vi "Tegam4040_Multi_Driver.vi"(9 "Input":dbl, 10 "Function":T1(ring), 11 "VISA Tegam4040":refnum<visa-resource-name>="PXI4::12::INSTR") -> (0 "error out":errorcluster)   [LabVIEW 2010]
uses:
  <instrlib>/Tegam4040/Tegam4040.lvlib
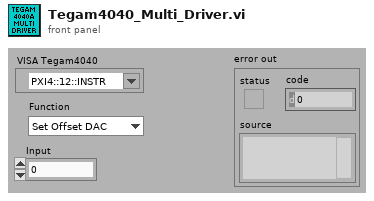
[diagram p1: front panel]
types:
  T1 = enum16{"Set Offset DAC", "Set Coupling (0=DC, 1=AC)", "Set Input (0=1M,1=50ohms)", "Set Atten (0-3=Open,1,10,100)", "Set Gain (0-2=1,10,100)"}
  T2 = enum16{"Attenuator Stage open", "Attenuation of 1", "Attenuation of 10", "Attenuation of 100"}
  T3 = enum16{"Disable Calibration", "Enable Calibration"}
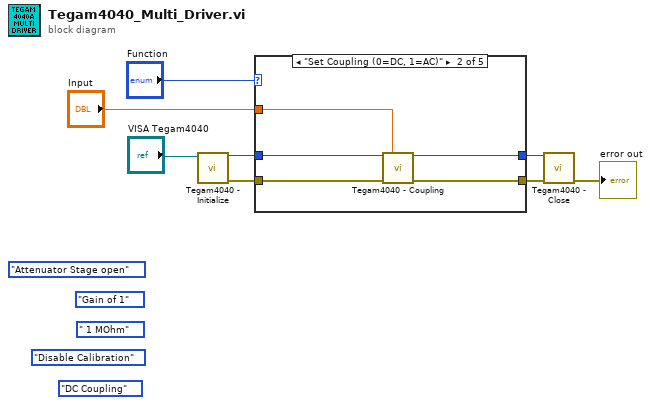
[diagram p0: block diagram]
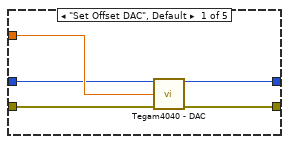
[diagram p2: hidden frame]
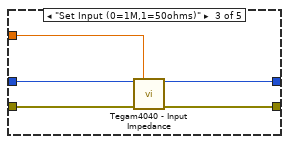
[diagram p3: hidden frame]
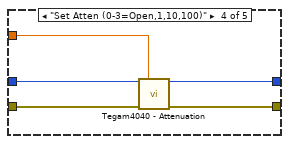
[diagram p4: hidden frame]
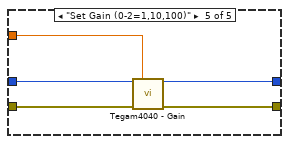
[diagram p5: hidden frame]
diagram:
  (unwired) T2."Attenuator Stage open" ("Attenuation")
  (unwired) enum16{"Gain of 1", "Gain of 10", "Gain of 100"}."Gain of 1" ("Gain")
  (unwired) enum16{" 1 MOhm", "50 Ohm"}." 1 MOhm" ("Input Impedance")
  (unwired) T3."Disable Calibration" ("Calibration")
  (unwired) enum16{"DC Coupling", "AC Coupling"}."DC Coupling" ("Coupling")
  n1 = call <instrlib>:"Tegam4040 - Initialize.vi"("VISA Tegam4040"="VISA Tegam4040") -> ("error out"=w7:errorcluster, "Instrument Session Handle"=w2:u32)  [unwired: 9 in]
  n2 = case shown="\"Set Coupling (0=DC, 1=AC)\"" "Function" {
    tunnel: w7 -> [w13 w17 w22 w28 w32]
    tunnel: [w12 w18 w23 w27 w33] -> w6
    tunnel: "Input" -> [w11 w14 w19 w24 w29]
    tunnel: w2 -> [w10 w16 w20 w26 w31]
    tunnel: [w9 w15 w21 w25 w30] -> w1
    frame "Set Offset DAC", Default {
      n3 = call <instrlib>:"Tegam4040 - DAC.vi"("Instrument Session Handle In"=w10, "DAC"=w11, "error in (no error)"=w13) -> ("Instrument Session Handle Out (dupl)"=w9:u32, "error out"=w12:errorcluster)  [unwired: 11 in]
    }
    frame "Set Coupling (0=DC, 1=AC)" {
      n4 = call <instrlib>:"Tegam4040 - Coupling.vi"("Instrument Session Handle In"=w16, "Coupling"=w14, "error in (no error)"=w17) -> ("Instrument Session Handle Out (dupl)"=w15:u32, "error out"=w18:errorcluster)  [unwired: 11 in]
    }
    frame "Set Input (0=1M,1=50ohms)" {
      n5 = call <instrlib>:"Tegam4040 - Input Impedance.vi"("Instrument Session Handle In"=w20, "Input Impedance"=w19, "error in (no error)"=w22) -> ("Instrument Session Handle Out (dupl)"=w21:u32, "error out"=w23:errorcluster)  [unwired: 11 in]
    }
    frame "Set Atten (0-3=Open,1,10,100)" {
      n6 = call <instrlib>:"Tegam4040 - Attenuation.vi"("Instrument Session Handle In"=w26, "Attenuation"=w24, "error in (no error)"=w28) -> ("Instrument Session Handle Out (dupl)"=w25:u32, "error out"=w27:errorcluster)  [unwired: 11 in]
    }
    frame "Set Gain (0-2=1,10,100)" {
      n7 = call <instrlib>:"Tegam4040 - Gain.vi"("Instrument Session Handle In"=w31, "Gain"=w29, "error in (no error)"=w32) -> ("Instrument Session Handle Out (dupl)"=w30:u32, "error out"=w33:errorcluster)  [unwired: 11 in]
    }
  }
  n8 = call <instrlib>:"Tegam4040 - Close.vi"("error in (no error)"=w6, "Instrument Session Handle"=w1) -> ("error out"=→"error out":errorcluster)  [unwired: 9 in]
